vi "get_subsystem_data.vi"(7 "Subsystem name":string, 8 "Double channel names":string[](array[string]), 9 "Boolean channel names":string[](array[string]), 10 "DBL Data":dbl[](array[numeric]), 11 "Bool Data":bool[](array[boolean])) -> (3 "Subsystem data out":T1={"Subsystem name"="Drive", "Double data points"=[], "Boolean data points"=[], "Boolean channel names"=[], "Double channel names"=[]})   [LabVIEW 2017, in "labview-standard-library.lvlib"]
uses:
  labview-standard-library.lvlib
  Subsystem_data.ctl
panel:
  in  "Subsystem data":T1={"Subsystem name"="Drive", "Double data points"=[], "Boolean data points"=[], "Boolean channel names"=[], "Double channel names"=[]}
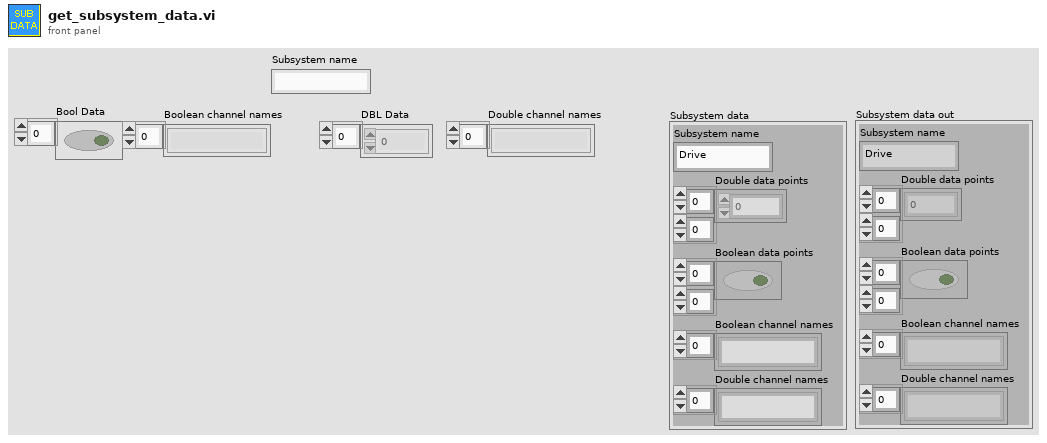
[diagram p1: front panel]
types:
  T1 = typedef "labview-standard-library.lvlib/Subsystem_data.ctl" = cluster{"Subsystem name":string, "Double data points":dbl[][], "Boolean data points":bool[][], "Boolean channel names":string[], "Double channel names":string[]}
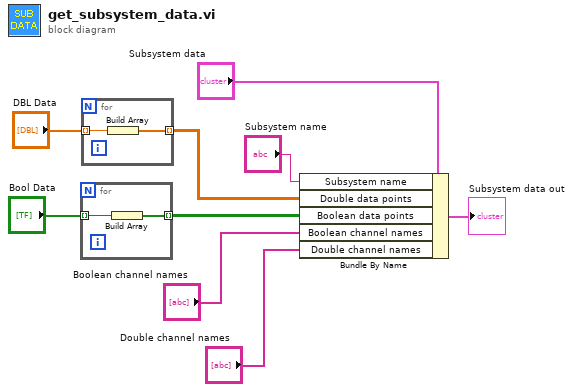
[diagram p0: block diagram]
diagram:
  n1 = for {
    tunnel: "Bool Data" -> [w11] mode=indexing
    tunnel: [w10] -> w4 mode=indexing
    n2 = Build Array(w11) -> (w10:bool[])
  }
  n3 = for {
    tunnel: "DBL Data" -> [w13] mode=indexing
    tunnel: [w12] -> w5 mode=indexing
    n4 = Build Array(w13) -> (w12:dbl[])
  }
  n5 = Bundle By Name(cluster="Subsystem data", "Subsystem name"="Subsystem name", "Double data points"=w5, "Boolean data points"=w4, "Boolean channel names"="Boolean channel names", "Double channel names"="Double channel names") -> (→"Subsystem data out":T1)
